vi "Control Panel.vi"() -> ()   [LabVIEW 2015]
uses:
  <vilib>/vision/NI_Vision_Development_Module.lvlib
panel:
  out "OCR ORIG 2":T1(plugin-control)
  out "OCR'd 2":T1(plugin-control)
  in  "File Path":path
  out "Read String":string
  out "Number of Matches (Color Pattern Matching 1) 2":i32
  out "Number of Matches (Color Pattern Matching 1)":i32
  in  "stop 5":bool
  out "Image 7":T1(plugin-control)
  in  "Contrast::Mode 3":u32(ring)=2 items=["Manual"=2]
  in  "Contrast::Value 3":dbl=0.13 min=0.0 max=0.3
  out "Green":T2(array[cluster]) {"Bounding Box"."y" format="%.2f"; "Bounding Box"."x" format="%.2f"; "Position"."y" format="%.2f"; "Position"."x" format="%.2f"; "Score" format="%.2f"; "Scale" format="%.2f"; "Angle" format="%.2f"}
  in  "stop 4":bool
  out "Image 6":T1(plugin-control)
  in  "Contrast::Mode 2":u32(ring)=2 items=["Manual"=2]
  in  "Contrast::Value 2":dbl=0.13 min=0.0 max=0.3
  out "Red":T2(array[cluster]) {"Bounding Box"."y" format="%.2f"; "Bounding Box"."x" format="%.2f"; "Position"."y" format="%.2f"; "Position"."x" format="%.2f"; "Score" format="%.2f"; "Scale" format="%.2f"; "Angle" format="%.2f"}
  in  "stop 3":bool
  out "OCR ORIG":T1(plugin-control)
  in  "Contrast::Mode":u32(ring)=2 items=["Manual"=2]
  in  "Contrast::Value":dbl=0.13 min=0.0 max=0.3
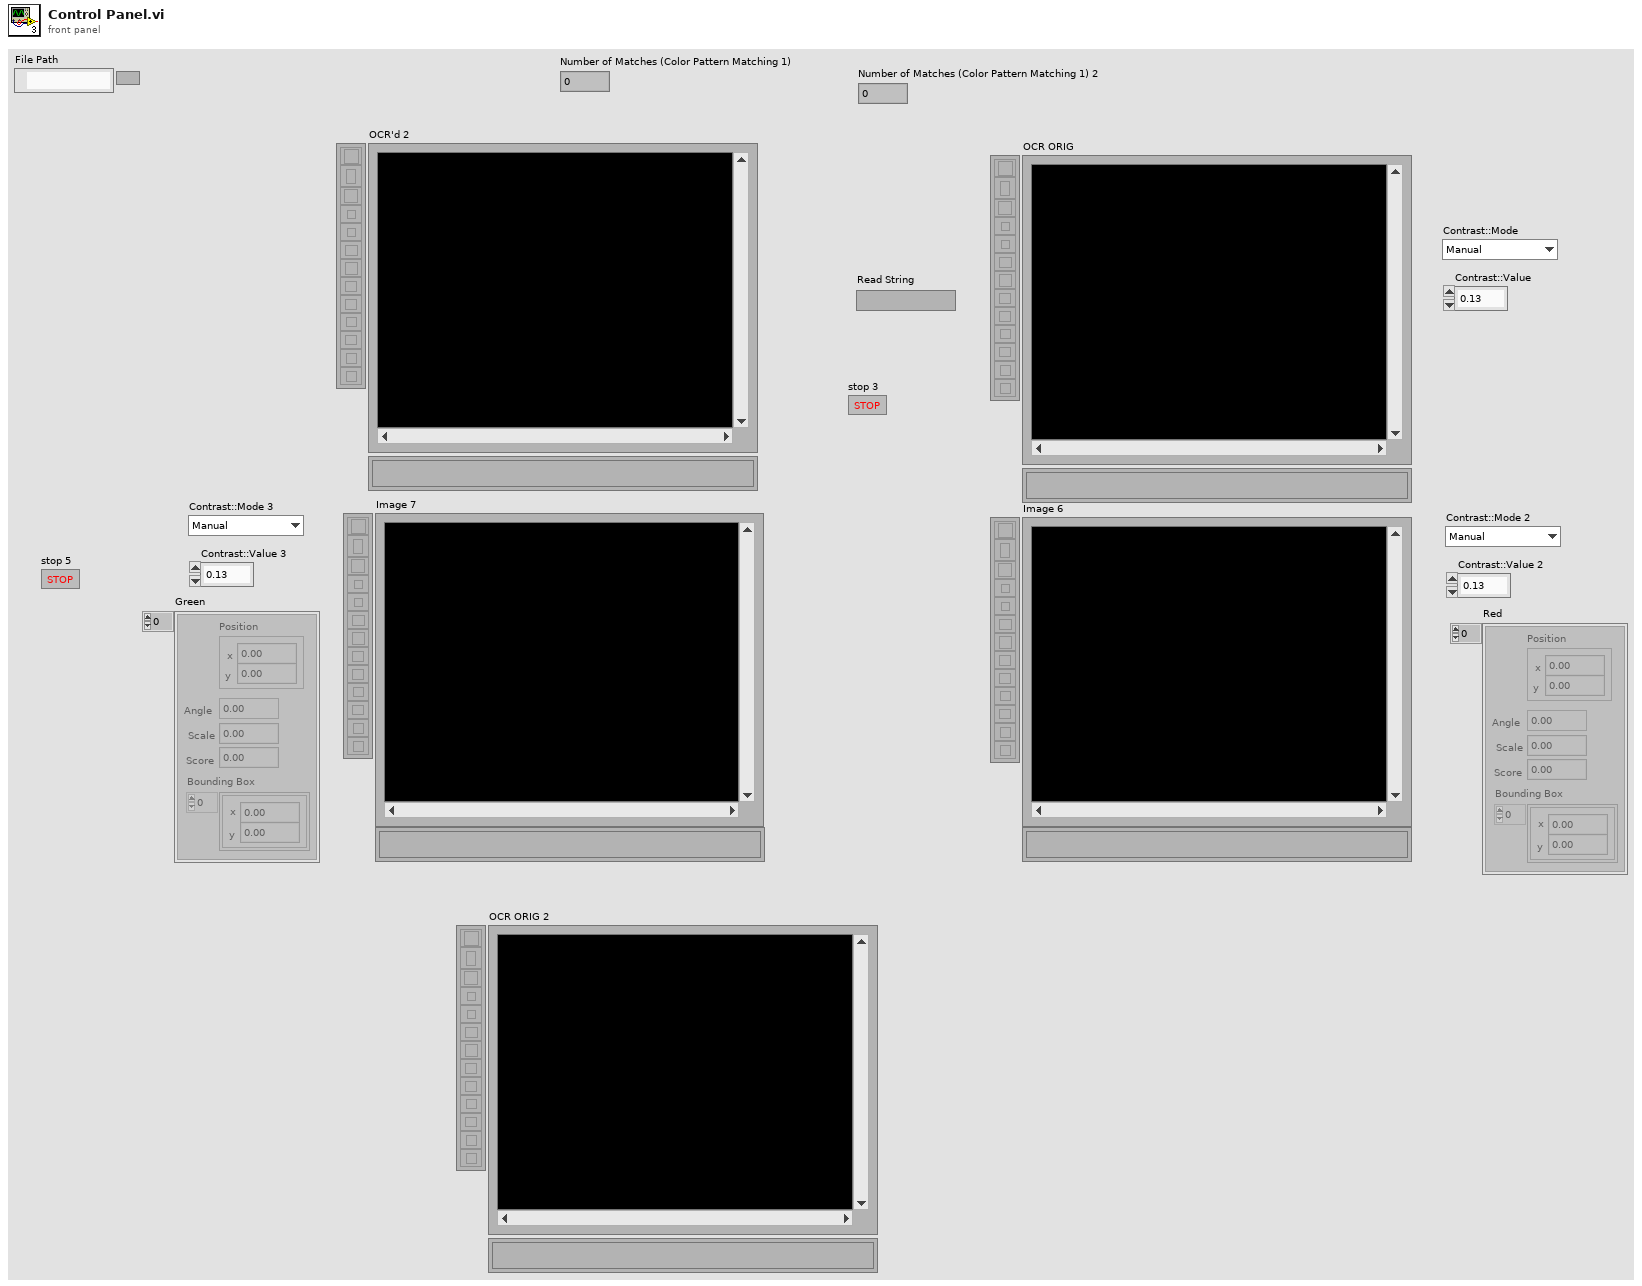
[diagram p1: front panel]
types:
  T1 = typedef "IMAQ Image.ctl" = refnum<image>
  T2 = cluster{"Position":cluster{"x":sgl, "y":sgl}, "Angle":sgl, "Scale":sgl, "Score":sgl, "Bounding Box":cluster{"x":sgl, "y":sgl}[]}[]
  T3 = typedef "IMAQ Rectangle" = cluster{"Left":i32, "Top":i32, "Right":i32, "Bottom":i32, "Rotation":dbl}
  T4 = cluster{"Reference System":cluster{"Origin":cluster{"X":sgl, "Y":sgl}, "Angle (deg)":sgl, "Axis Reference":u32}, "Measurement System":cluster{"Origin":cluster{"X":sgl, "Y":sgl}, "Angle (deg)":sgl, "Axis Reference":u32}}
  T5 = typedef "IMAQ OCR Session.ctl" = refnum<k1>
  T6 = typedef "ROI Descriptor" = cluster{"Global Rectangle":i32[], "Contours":cluster{"ID":enum32{"External", "Internal"}, "Type":u32, "Coordinates":i32[]}[]}
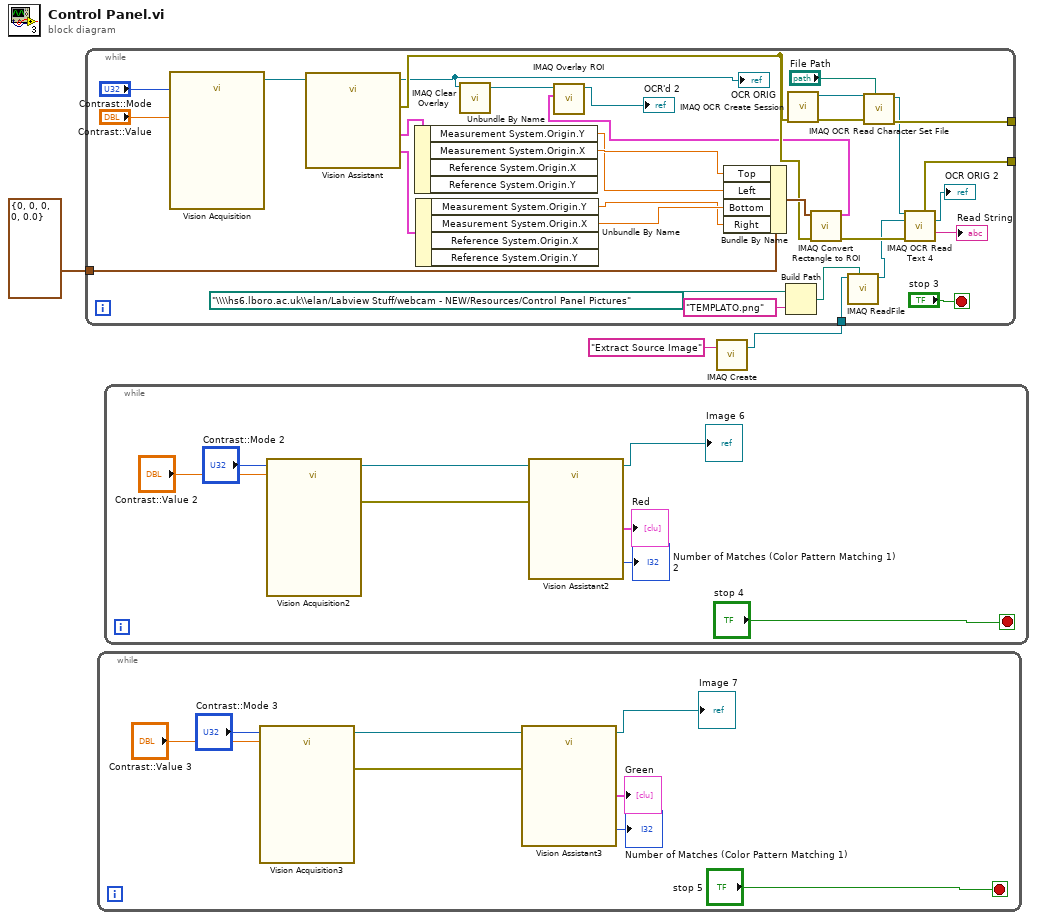
[diagram p0: block diagram]
diagram:
  n1 = while {
    stop <- "stop 5" stop-if-true
    n2 = call "Vision Acquisition3"("Contrast::Mode"="Contrast::Mode 3", "Contrast::Value"="Contrast::Value 3") -> ("Image Out"=w10:T1, "error out"=w9:errorcluster)  [unwired: 22 in, 2 out]
    n3 = call "Vision Assistant3"("Image In"=w10, "error in"=w9) -> ("Image Out"=→"Image 7":T1, "Matches (Color Pattern Matching 1)"=→"Green":T2, "Number of Matches (Color Pattern Matching 1)"=→"Number of Matches (Color Pattern Matching 1)":i32)  [unwired: 21 in, 2 out]
  }
  n4 = while {
    stop <- "stop 4" stop-if-true
    n5 = call "Vision Acquisition2"("Contrast::Mode"="Contrast::Mode 2", "Contrast::Value"="Contrast::Value 2") -> ("Image Out"=w18:T1, "error out"=w17:errorcluster)  [unwired: 22 in, 2 out]
    n6 = call "Vision Assistant2"("Image In"=w18, "error in"=w17) -> ("Image Out"=→"Image 6":T1, "Matches (Color Pattern Matching 1)"=→"Red":T2, "Number of Matches (Color Pattern Matching 1)"=→"Number of Matches (Color Pattern Matching 1) 2":i32)  [unwired: 21 in, 2 out]
  }
  n7 = call "IMAQ Create"("Image Name"="Extract Source Image") -> ("New Image"=w1:T1)  [unwired: 4 in, 1 out]
  n8 = while {
    tunnel: T3 {"Left"=0, "Top"=0, "Right"=0, "Bottom"=0, "Rotation"=0.0} ("Rectangle") -> [w40]
    tunnel: [w34] -> _
    tunnel: [w33] -> _
    tunnel: w1 -> [w25]
    stop <- "stop 3" stop-if-true
    n9 = call "Vision Acquisition"("Contrast::Mode"="Contrast::Mode", "Contrast::Value"="Contrast::Value") -> ("Image Out"=w22:T1)  [unwired: 22 in, 3 out]
    n10 = call "Vision Assistant"("Image In"=w22) -> ("Image Out"=w20:T1, "Coordinate System Out (TOP LEFT COORD)"=w47:T4, "Coordinate System Out (BOTTOM RIGHT COORD)"=w46:T4, "error out"=w36:errorcluster)  [unwired: 23 in]
    "OCR ORIG" <- w20
    n11 = Unbundle By Name(w47) -> ("Measurement System.Origin.Y"=w44:sgl, "Measurement System.Origin.X"=w45:sgl)  [unwired: 2 out]
    n12 = Unbundle By Name(w46) -> ("Measurement System.Origin.Y"=w42:sgl, "Measurement System.Origin.X"=w43:sgl)  [unwired: 2 out]
    n13 = call "IMAQ Clear Overlay"("Image"=w20) -> ("Image Out"=w29:T1)  [unwired: 2 in, 8 out]
    n14 = Bundle By Name(cluster=w40, "Top"=w45, "Left"=w44, "Bottom"=w43, "Right"=w42) -> (w41:T3)
    n15 = Build Path(base path=path "\\\\hs6.lboro.ac.uk\\elan/Labview Stuff/webcam - NEW/Resources/Control Panel Pictures", name or relative path="TEMPLATO.png") -> (appended path=w24:path)
    n16 = call "IMAQ OCR Create Session"("error in (no error)"=w36) -> ("error out"=w37:errorcluster, "IMAQ OCR Session"=w32:T5)  [unwired: 9 in]
    n17 = call "IMAQ Convert Rectangle to ROI"("error in (no error)"=w36, "Rectangle"=w41) -> ("error out"=w35:errorcluster, "ROI Descriptor"=w28:T6)  [unwired: 7 in]
    n18 = call "IMAQ Overlay ROI"("ROI Descriptor"=w28, "Image"=w29) -> ("Image Out"=→"OCR'd 2":T1)  [unwired: 4 in, 5 out]
    n19 = call "IMAQ ReadFile"("File Path"=w24, "Image"=w25) -> ("Image Out"=w21:T1)  [unwired: 5 in, 4 out]
    n20 = call "IMAQ OCR Read Character Set File"("File Path"="File Path", "error in (no error)"=w37, "IMAQ OCR Session"=w32) -> ("error out"=w33:errorcluster, "IMAQ OCR Session (dup)"=w31:T5)  [unwired: 6 in, 1 out]
    n21 = call "IMAQ OCR Read Text 4"("IMAQ OCR Session"=w31, "Image"=w21, "error in (no error)"=w35) -> ("Image (dup)"=→"OCR ORIG 2":T1, "Read String"=→"Read String":string, "error out"=w34:errorcluster)  [unwired: 6 in, 4 out]
  }
